vi "Read From File.vi"(8 "error in":errorcluster, 11 "file path":path) -> (0 "error out":errorcluster, 2 "text":string)   [LabVIEW 2020, in "CICD.lvlib"]
uses:
  CICD.lvlib
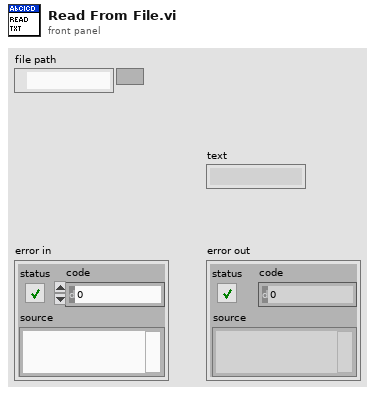
[diagram p1: front panel]
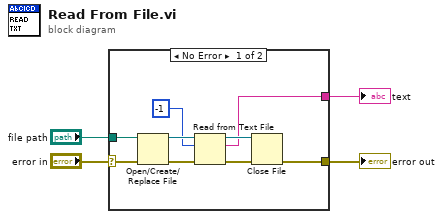
[diagram p0: block diagram]
diagram:
  n1 = case shown="No Error" "error in" {
    selector: "error in" -> [w5 w14]
    tunnel: [w11 w14] -> w4
    tunnel: [w7 _] -> w3
    tunnel: "file path" -> [w6 _]
    frame No Error {
      n2 = Open/Create/Replace File(file path (use dialog)=w6, error in=w5) -> (refnum out=w9:refnum<file>, error out=w12:errorcluster)  [unwired: 4 in, 1 out]
      n3 = Read from Text File(file (use dialog)=w9, count=-1, error in=w12) -> (refnum out=w10:refnum<file>, text=w7:string, error out=w13:errorcluster)  [unwired: 1 in, 1 out]
      n4 = Close File(refnum=w10, error in=w13) -> (error out=w11:errorcluster)  [unwired: 1 out]
    }
    frame Error {
    }
  }
  "error out" <- w4
  "text" <- w3
